vi "SaveConfiguration.vi"(10 "Matrix Cfg":T1={"Other Outputs"={"Alarm"=FALSE, "Heater"=FALSE}, "CO2 Settings"={"Run C1"={"A-1,  1"=0.0, "A-3,  2"=0.0, "A-4, 3"=0.0, "A-5, 4"=0.0, "ABCD-7, 5"=0.0, "A-8, 6"=0.0, "B-1,  7"=0.0, "B-3, 8"=0.0, "B-4,  9"=0.0, "B-5, 10"=0.0, "B-8, 11"=0.0, "C-1, 12"=0.0, "C-3, 13"=0.0, "C-4, 14"=0.0, "C-5,  15"=0.0, "C-8, 16"=0.0, "D-1, 17"=0.0, "D-3, 18"=0.0, "D-4,  19"=0.0, "D-5,  20"=0.0, "D-8,  21"=0.0}, "Run C2"={"A-1,  1"=0.0, "A-3,  2"=0.0, "A-4, 3"=0.0, "A-5, 4"=0.0, "ABCD-7, 5"=0.0, "A-8, 6"=0.0, "B-1,  7"=0.0, "B-3, 8"=0.0, "B-4,  9"=0.0, "B-5, 10"=0.0, "B-8, 11"=0.0, "C-1, 12"=0.0, "C-3, 13"=0.0, "C-4, 14"=0.0, "C-5,  15"=0.0, "C-8, 16"=0.0, "D-1, 17"=0.0, "D-3, 18"=0.0, "D-4,  19"=0.0, "D-5,  20"=0.0, "D-8,  21"=0.0}, "Hold C3"={"A-1,  1"=0.0, "A-3,  2"=0.0, "A-4, 3"=0.0, "A-5, 4"=0.0, "ABCD-7, 5"=0.0, "A-8, 6"=0.0, "B-1,  7"=0.0, "B-3, 8"=0.0, "B-4,  9"=0.0, "B-5, 10"=0.0, "B-8, 11"=0.0, "C-1, 12"=0.0, "C-3, 13"=0.0, "C-4, 14"=0.0, "C-5,  15"=0.0, "C-8, 16"=0.0, "D-1, 17"=0.0, "D-3, 18"=0.0, "D-4,  19"=0.0, "D-5,  20"=0.0, "D-8,  21"=0.0}, "Hold C4"={"A-1,  1"=0.0, "A-3,  2"=0.0, "A-4, 3"=0.0, "A-5, 4"=0.0, "ABCD-7, 5"=0.0, "A-8, 6"=0.0, "B-1,  7"=0.0, "B-3, 8"=0.0, "B-4,  9"=0.0, "B-5, 10"=0.0, "B-8, 11"=0.0, "C-1, 12"=0.0, "C-3, 13"=0.0, "C-4, 14"=0.0, "C-5,  15"=0.0, "C-8, 16"=0.0, "D-1, 17"=0.0, "D-3, 18"=0.0, "D-4,  19"=0.0, "D-5,  20"=0.0, "D-8,  21"=0.0}, "High CO2 Forces"={"A-1, 1"=FALSE, "A-3, 2"=FALSE, "A-4, 3"=FALSE, "A-5, 4"=FALSE, "ABCD-7, 5"=FALSE, "A-8, 6"=FALSE, "B-1,  7"=FALSE, "B-3, 8"=FALSE, "B-4, 9"=FALSE, "B-5, 10"=FALSE, "B-8,  11"=FALSE, "C-1, 12"=FALSE, "C-3, 13"=FALSE, "C-4,  14"=FALSE, "C-5,  15"=FALSE, "C-8, 16"=FALSE, "D-1, 17"=FALSE, "D-3, 18"=FALSE, "D-4, 19"=FALSE, "D-5,  20"=FALSE, "D-8,  21"=FALSE}}, "AD Settings"={"Set Point Force"={"A-1,  1"=0.0, "A-3,  2"=0.0, "A-4, 3"=0.0, "A-5, 4"=0.0, "ABCD-7, 5"=0.0, "A-8, 6"=0.0, "B-1,  7"=0.0, "B-3, 8"=0.0, "B-4,  9"=0.0, "B-5, 10"=0.0, "B-8, 11"=0.0, "C-1, 12"=0.0, "C-3, 13"=0.0, "C-4, 14"=0.0, "C-5,  15"=0.0, "C-8, 16"=0.0, "D-1, 17"=0.0, "D-3, 18"=0.0, "D-4,  19"=0.0, "D-5,  20"=0.0, "D-8,  21"=0.0}, "Run A1"={"A-1,  1"=0.0, "A-3,  2"=0.0, "A-4, 3"=0.0, "A-5, 4"=0.0, "ABCD-7, 5"=0.0, "A-8, 6"=0.0, "B-1,  7"=0.0, "B-3, 8"=0.0, "B-4,  9"=0.0, "B-5, 10"=0.0, "B-8, 11"=0.0, "C-1, 12"=0.0, "C-3, 13"=0.0, "C-4, 14"=0.0, "C-5,  15"=0.0, "C-8, 16"=0.0, "D-1, 17"=0.0, "D-3, 18"=0.0, "D-4,  19"=0.0, "D-5,  20"=0.0, "D-8,  21"=0.0}, "Run A2"={"A-1,  1"=0.0, "A-3,  2"=0.0, "A-4, 3"=0.0, "A-5, 4"=0.0, "ABCD-7, 5"=0.0, "A-8, 6"=0.0, "B-1,  7"=0.0, "B-3, 8"=0.0, "B-4,  9"=0.0, "B-5, 10"=0.0, "B-8, 11"=0.0, "C-1, 12"=0.0, "C-3, 13"=0.0, "C-4, 14"=0.0, "C-5,  15"=0.0, "C-8, 16"=0.0, "D-1, 17"=0.0, "D-3, 18"=0.0, "D-4,  19"=0.0, "D-5,  20"=0.0, "D-8,  21"=0.0}, "Hold A3"={"A-1,  1"=0.0, "A-3,  2"=0.0, "A-4, 3"=0.0, "A-5, 4"=0.0, "ABCD-7, 5"=0.0, "A-8, 6"=0.0, "B-1,  7"=0.0, "B-3, 8"=0.0, "B-4,  9"=0.0, "B-5, 10"=0.0, "B-8, 11"=0.0, "C-1, 12"=0.0, "C-3, 13"=0.0, "C-4, 14"=0.0, "C-5,  15"=0.0, "C-8, 16"=0.0, "D-1, 17"=0.0, "D-3, 18"=0.0, "D-4,  19"=0.0, "D-5,  20"=0.0, "D-8,  21"=0.0}, "Hold A4"={"A-1,  1"=0.0, "A-3,  2"=0.0, "A-4, 3"=0.0, "A-5, 4"=0.0, "ABCD-7, 5"=0.0, "A-8, 6"=0.0, "B-1,  7"=0.0, "B-3, 8"=0.0, "B-4,  9"=0.0, "B-5, 10"=0.0, "B-8, 11"=0.0, "C-1, 12"=0.0, "C-3, 13"=0.0, "C-4, 14"=0.0, "C-5,  15"=0.0, "C-8, 16"=0.0, "D-1, 17"=0.0, "D-3, 18"=0.0, "D-4,  19"=0.0, "D-5,  20"=0.0, "D-8,  21"=0.0}, "High AD Diff "={"A-1, 1"=FALSE, "A-3, 2"=FALSE, "A-4, 3"=FALSE, "A-5, 4"=FALSE, "ABCD-7, 5"=FALSE, "A-8, 6"=FALSE, "B-1,  7"=FALSE, "B-3, 8"=FALSE, "B-4, 9"=FALSE, "B-5, 10"=FALSE, "B-8,  11"=FALSE, "C-1, 12"=FALSE, "C-3, 13"=FALSE, "C-4,  14"=FALSE, "C-5,  15"=FALSE, "C-8, 16"=FALSE, "D-1, 17"=FALSE, "D-3, 18"=FALSE, "D-4, 19"=FALSE, "D-5,  20"=FALSE, "D-8,  21"=FALSE}, "Delay S"={"A-1,  1"=0.0, "A-3,  2"=0.0, "A-4, 3"=0.0, "A-5, 4"=0.0, "ABCD-7, 5"=0.0, "A-8, 6"=0.0, "B-1,  7"=0.0, "B-3, 8"=0.0, "B-4,  9"=0.0, "B-5, 10"=0.0, "B-8, 11"=0.0, "C-1, 12"=0.0, "C-3, 13"=0.0, "C-4, 14"=0.0, "C-5,  15"=0.0, "C-8, 16"=0.0, "D-1, 17"=0.0, "D-3, 18"=0.0, "D-4,  19"=0.0, "D-5,  20"=0.0, "D-8,  21"=0.0}}, "Max Altitude"=0.0, "DefaultLocation"=path "", "COM Parameters"={"Port"="", "Baud Rate"=0, "Data Bits"=0, "Parity"=0, "Stop Bits"=0, "Flow Control"=0}, "AltUnits"=FALSE, "AltCalc"=FALSE, "Mode"=enum."Stby", "Channel Names"={"A-1,  1"="Main", "A-3,  2"="Main", "A-4, 3"="Recirculation", "A-5, 4"="Scrubber", "ABCD-7, 5"="Oxygen", "D-8, 6"="Vent", "B-1,  7"="Boost A", "B-3, 8"="Boost A", "B-4,  9"="Recirculation", "B-5, 10"="Scrubber", "B-8, 11"="Vent", "C-1, 12"="Boost B", "C-3, 13"="Boost B", "C-4, 14"="Recirculation", "C-5,  15"="Scrubber", "C-8, 16"="Vent", "D-1, 17"="+24V", "D-3, 18"="Main", "D-4,  19"="Boost A", "D-5,  20"="Boost B", "D-8,  21"="Vent"}, "Setpoint"=0.0} {"COM Parameters"."Flow Control" items=["None"=0, "XON/XOFF"=1, "RTS/CTS"=2, "DTR/DSR"=4]; "COM Parameters"."Stop Bits" items=["1.0"=10, "1.5"=15, "2.0"=20]; "COM Parameters"."Parity" items=["None", "Odd", "Even", "Mark", "Space"]; "COM Parameters"."Data Bits" min=5 max=8 step=1}, 11 "file":path) -> ()   [LabVIEW 2012]
uses:
  Type Defs/CfgData.ctl
  Type Defs/CO2 Settings.ctl
  Type Defs/Output Values.ctl
  Type Defs/Output Switches.ctl
  Type Defs/AD Settings.ctl
  Type Defs/Named Final Output name list ordered.ctl
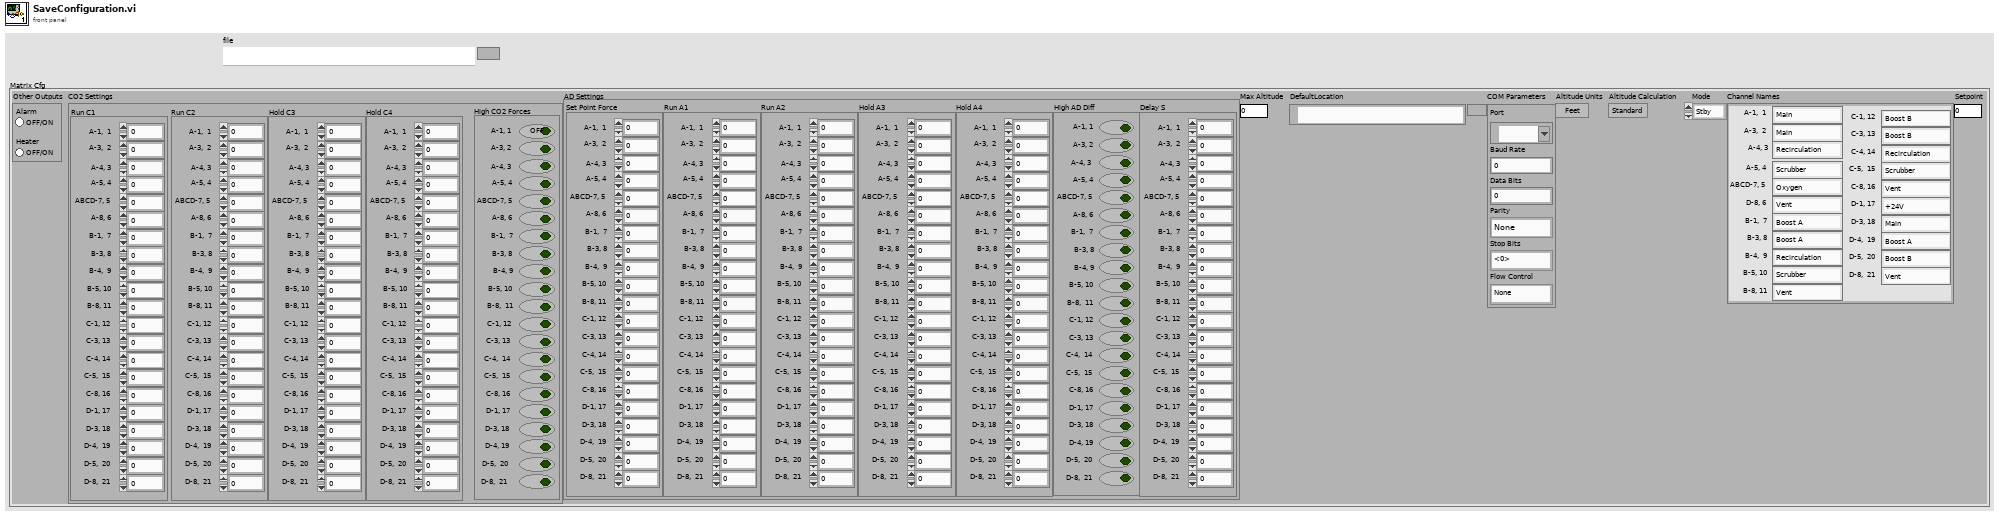
[diagram p1: front panel]
types:
  T1 = typedef "CfgData.ctl" = cluster{"Other Outputs":cluster{"Alarm":bool, "Heater":bool}, "CO2 Settings":T2, "AD Settings":T5, "Max Altitude":sgl, "DefaultLocation":path, "COM Parameters":cluster{"Port":refnum<visa-resource-name>, "Baud Rate":u32, "Data Bits":u16, "Parity":u16, "Stop Bits":u16, "Flow Control":u16}, "AltUnits":bool, "AltCalc":bool, "Mode":enum8{"Off", "Stby", "Hold", "Run"}, "Channel Names":T6, "Setpoint":sgl}
  T2 = typedef "CO2 Settings.ctl" = cluster{"Run C1":T3, "Run C2":T3, "Hold C3":T3, "Hold C4":T3, "High CO2 Forces":T4}
  T3 = typedef "Output Values.ctl" = cluster{"A-1,  1":dbl, "A-3,  2":dbl, "A-4, 3":dbl, "A-5, 4":dbl, "ABCD-7, 5":dbl, "A-8, 6":dbl, "B-1,  7":dbl, "B-3, 8":dbl, "B-4,  9":dbl, "B-5, 10":dbl, "B-8, 11":dbl, "C-1, 12":dbl, "C-3, 13":dbl, "C-4, 14":dbl, "C-5,  15":dbl, "C-8, 16":dbl, "D-1, 17":dbl, "D-3, 18":dbl, "D-4,  19":dbl, "D-5,  20":dbl, "D-8,  21":dbl}
  T4 = typedef "Output Switches.ctl" = cluster{"A-1, 1":bool, "A-3, 2":bool, "A-4, 3":bool, "A-5, 4":bool, "ABCD-7, 5":bool, "A-8, 6":bool, "B-1,  7":bool, "B-3, 8":bool, "B-4, 9":bool, "B-5, 10":bool, "B-8,  11":bool, "C-1, 12":bool, "C-3, 13":bool, "C-4,  14":bool, "C-5,  15":bool, "C-8, 16":bool, "D-1, 17":bool, "D-3, 18":bool, "D-4, 19":bool, "D-5,  20":bool, "D-8,  21":bool}
  T5 = typedef "AD Settings.ctl" = cluster{"Set Point Force":T3, "Run A1":T3, "Run A2":T3, "Hold A3":T3, "Hold A4":T3, "High AD Diff ":T4, "Delay S":T3}
  T6 = typedef "Named Final Output name list ordered.ctl" = cluster{"A-1,  1":string, "A-3,  2":string, "A-4, 3":string, "A-5, 4":string, "ABCD-7, 5":string, "D-8, 6":string, "B-1,  7":string, "B-3, 8":string, "B-4,  9":string, "B-5, 10":string, "B-8, 11":string, "C-1, 12":string, "C-3, 13":string, "C-4, 14":string, "C-5,  15":string, "C-8, 16":string, "D-1, 17":string, "D-3, 18":string, "D-4,  19":string, "D-5,  20":string, "D-8,  21":string}
  T7 = enum16{"open", "replace", "create", "open or create", "replace or create", "replace or create with confirmation"}
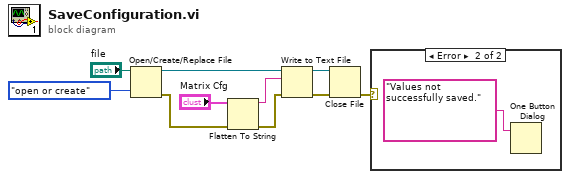
[diagram p0: block diagram]
diagram:
  n1 = Open/Create/Replace File(file path (use dialog)="file", operation (0:open)=T7."open or create") -> (refnum out=w3:refnum<file>, error out=w2:errorcluster)  [unwired: 4 in, 1 out]
  n2 = Flatten To String(anything="Matrix Cfg", error in (no error)=w2) -> (data string=w6:string, error out=w10:errorcluster)  [unwired: 2 in, 1 out]
  n3 = Write to Text File(file (use dialog)=w3, text=w6, error in=w10) -> (refnum out=w7:refnum<file>, error out=w8:errorcluster)  [unwired: 1 in, 1 out]
  n4 = Close File(refnum=w7, error in=w8) -> (error out=w9:errorcluster)  [unwired: 1 out]
  n5 = case shown="Error" w9 {
    frame No Error {
    }
    frame Error {
      n6 = One Button Dialog(message="Values not successfully saved.") -> ()  [unwired: 1 in, 1 out]
    }
  }
